vi "4.4.vi"() -> ()   [LabVIEW 2017]
panel:
  in  "实时温度":dbl
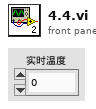
[diagram p1: front panel]
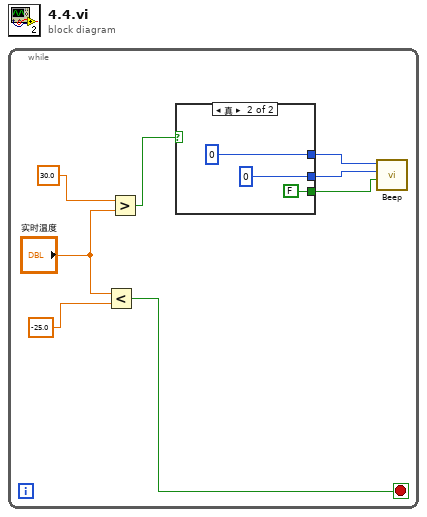
[diagram p0: block diagram]
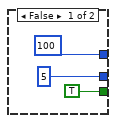
[diagram p2: hidden frame]
diagram:
  n1 = while {
    stop <- w5 stop-if-true
    n2 = Less?(x="实时温度", y=-25.0) -> (x < y?=w5:bool)
    n3 = Greater?(x=30.0, y="实时温度") -> (0:w6:bool)
    n4 = case shown="真" w6 {
      tunnel: [100 0] -> w4
      tunnel: [5 0] -> w3
      tunnel: [TRUE ("use system alert? (T)") FALSE ("use system alert? (T)")] -> w1
      frame False {
      }
      frame True {
      }
    }
    n5 = call <vilib>:"Beep.vi"("use system alert? (T)"=w1, "duration (msec)"=w3, "frequency (Hz)"=w4) -> ()  [unwired: 9 in]
  }
